vi "nanocal -- nuclear schottky fit V7.vi"() -> ()   [LabVIEW 2021] (continued)
                  n129 = Generate User Event(user event=w300, event data cluster="interface: update circle fit plot" ("event data")) -> (user event out=w295:refnum<user-event>)  [unwired: 2 in, 1 out]
                  n130 = Generate User Event(user event=w295, event data cluster="interface: update curvature plot" ("event data")) -> ()  [unwired: 2 in, 2 out]
                }
              }
              n131 = call "nanocal -- gradient descent.vi"("# steps"="#grad steps", "action"=nanocal_--_gradient_descent_--_action."step", "newton pars"=w288, "parameter keys IN"=w289, "parameter Map IN"=w283, "factors Map IN"=w282) -> ("logarithmic derivatives OUT"=w284:dbl[], "step factors OUT"=w291:map{T2, dbl}, "R(ω) out"=w281:cdb[], "goodness OUT"=w271:dbl, "oscillations"=→"Plot: oscillations":cluster{"Array":i32[], "Array":dbl[]})  [unwired: 1 in]
              n132 = for {
                tunnel: w289 -> [w302] mode=indexing
                shift-right: [w306] -> _
                shift-left: w291 -> [w306]
                shift-right: [w304] -> w272
                shift-left: w283 -> [w305]
                n133 = Look In Map(map=w306, key=w302) -> (value=w303:dbl)  [unwired: 1 in, 1 out]
                n134 = in-place {
                  in-place-border: w303 -> [w308]
                  n135 = in-place-map #1(w305, w302) -> (w309:dbl)  [unwired: 1 in, 1 out]
                  n136 = Multiply(x=w308, y=w309) -> (x*y=w307:dbl)
                  n137 = in-place-map #1(w307) -> (w304:map{T2, dbl})  [unwired: 1 in, 2 out]
                }
              }
              n138 = Absolute Value(x=w284) -> (abs(x)=→"|v_i| = | dlogG/dlogα_i | (log scale slider)":dbl[])
              n139 = local write "vector v=dlogG/dlogα of logarithmic derivatives"(w284) -> ()
              n140 = local write "R(ω) fit out"(w281) -> ()
              n141 = local write "Goodness"(w271) -> ()
              n142 = local write "parameter map"(w272) -> ()
              "current step ind" <- w275
            }
            n143 = local write "newton is active"(w263) -> ()
            "current  ind" <- 0 ("plot ind")
          }
          frame "action: parse string" {
            n144 = local read "String"() -> (w323:string)
            n145 = Generate User Event(user event=w315, event data cluster="interface: update list from parameter map" ("event data")) -> ()  [unwired: 2 in, 2 out]
            n146 = call "string parse mathematica assosiated array.vi"("action"=mathematica_string_map_action."parse string" ("derivative"), "String in"=w323) -> ("Map OUT"=w317:map{T2, dbl})  [unwired: 8 in, 1 out]
            n147 = Generate User Event ("action User Event")(user event=w321, event data cluster="action: update state of selectors" ("event data")) -> (user event out=w318:refnum<user-event>)  [unwired: 2 in, 1 out]
            n148 = Generate User Event ("action User Event")(user event=w318, event data cluster="action: replot colors" ("event data")) -> ()  [unwired: 2 in, 2 out]
            n149 = local write "parameter map"(w317) -> ()
          }
          frame "action: read mathematica string" {
            w333 = map{string, path} {}  # Size: 0
            w348 = map{T2, dbl} {}  # Size: 0
            w345 = set{dbl} {}  # Size: 0
            w349 = map{string, map{T2, dbl}} {}  # Size: 0
            w339 = map{string, string} {}  # Size: 0
            n150 = local read "side map to STR"() -> (w341:map{T8, string})
            n151 = local read "side map to NUM"() -> (w340:map{T8, i32})
            n152 = local read "data file parameters map"() -> (w342:map{T2, T18})
            n153 = local read "file pattern"() -> (w336:string)
            n154 = local read "folder"() -> (w337:path)
            n155 = Generate User Event(user event=w346, event data cluster="action: update enums" ("event data")) -> ()  [unwired: 2 in, 2 out]
            n156 = call "string parse mathematica list assosiated array -- V2.vi"("action"=3-lorentzian-heat-response_action."parse string" ("derivative"), "string IN"="string IN") -> ("Map OUT"=w350:map{string, map{T2, dbl}})  [unwired: 8 in, 1 out]
            n157 = call <vilib>:"Recursive File List.vi"("pattern"=w336, "Continue Recursing on Error? (F)"=TRUE, "Folder Path"=w337) -> ("All Files in Dir"=w334:path[])  [unwired: 4 in, 4 out]
            n158 = for {
              tunnel: w334 -> [w358] mode=indexing
              shift-right: [w372] -> w324
              shift-left: w350 -> [w382]
              shift-right: [w369] -> w344
              shift-left: w339 -> [w381]
              shift-right: [w368] -> w343
              shift-left: w349 -> [w377]
              shift-right: [w379] -> w328
              shift-left: w345 -> [w371]
              shift-right: [w370] -> w327
              shift-left: w345 -> [w380]
              tunnel: w348 -> [w375]
              shift-right: [w365] -> w326
              shift-left: w345 -> [w378]
              shift-right: [w367] -> w329
              shift-left: w345 -> [w376]
              tunnel: w342 -> [w374]
              shift-right: [w366] -> w331
              shift-left: w345 -> [w373]
              tunnel: w340 -> [w363]
              tunnel: w341 -> [w362]
              shift-right: [w359] -> w338
              shift-left: w333 -> [w360]
              w361 = T8[] [enum."sam", enum."ref"] items=["sam", "ref"]
              n159 = Strip Path(path=w358) -> (name=w357:string)  [unwired: 1 out]
              n160 = call "filename-manage.vi"("filename-action"=filename-action."getIDStock", "file name IN"=w357) -> ("string OUT"=w364:string)  [unwired: 7 in, 2 out]
              n161 = for {
                tunnel: w374 -> [w408]
                tunnel: w357 -> [w385]
                tunnel: w364 -> [w397]
                shift-right: [w406] -> w372
                shift-left: w382 -> [w417]
                shift-right: [w412] -> w379
                shift-left: w371 -> [w405]
                shift-right: [w404] -> w370
                shift-left: w380 -> [w413]
                shift-right: [w398] -> w365
                shift-left: w378 -> [w411]
                shift-right: [w399] -> w367
                shift-left: w376 -> [w409]
                shift-right: [w400] -> w366
                shift-left: w373 -> [w407]
                shift-right: [w401] -> w368
                shift-left: w377 -> [w410]
                shift-right: [w402] -> w369
                shift-left: w381 -> [w416]
                tunnel: w363 -> [w390]
                tunnel: w375 -> [w395]
                tunnel: w362 -> [w392]
                tunnel: w361 -> [w389] mode=indexing
                shift-right: [w386] -> w359
                shift-left: w360 -> [w387]
                tunnel: w358 -> [w384]
                # "internal key"
                n162 = Look In Map(map=w392, key=w389) -> (value=w391:string)  [unwired: 1 in, 1 out]
                n163 = Look In Map(map=w390, key=w389) -> (value=w388:i32)  [unwired: 1 in, 1 out]
                n164 = Concatenate Strings(w397, w391) -> (w396:string)
                n165 = Insert Into Map(map in=w395, key=3-lorentzian-parameters."side (S|R)", value=w388) -> (map out=w394:map{T2, dbl})  [unwired: 2 out]
                n166 = for {
                  shift-right: [w423] -> w403
                  shift-left: w394 -> [w424]
                  tunnel: w408 -> [w422] mode=indexing
                  tunnel: w385 -> [w420]
                  n167 = Unbundle(w422) -> ("key"=w421:T2, "filename-action"=w419:T18)
                  n168 = call "filename-manage.vi"("filename-action"=w419, "file name IN"=w420) -> ("number OUT"=w418:dbl)  [unwired: 7 in, 2 out]
                  n169 = Insert Into Map(map in=w424, key=w421, value=w418) -> (map out=w423:map{T2, dbl})  [unwired: 2 out]
                }
                n170 = in-place {
                  in-place-border: [w466] -> w415
                  in-place-border: w403 -> [w465]
                  n171 = in-place-map #2(w417, w396) -> (w464:map{T2, dbl}, w466:bool)  [unwired: 1 in]
                  n172 = for {
                    tunnel: w465 -> [w472] mode=indexing
                    shift-right: [w470] -> w463
                    shift-left: w464 -> [w471]
                    n173 = Unbundle(w472) -> ("key"=w469:T2, "number OUT"=w468:dbl)
                    n174 = Insert Into Map(map in=w471, key=w469, value=w468) -> (map out=w470:map{T2, dbl})  [unwired: 2 out]
                  }
                  n175 = in-place-map #2(w463, LVMapReplaceAction."Modify Entry only if found" ("action")) -> (w406:map{string, map{T2, dbl}})  [unwired: 2 out]
                }
                n176 = Not(x=w415) -> (.not. x?=w414:bool)
                n177 = case shown="True" w414 {
                  tunnel: w416 -> [w432 w462]
                  tunnel: [w432 w461] -> w402
                  tunnel: w385 -> [_ w460]
                  tunnel: w396 -> [_ w434]
                  tunnel: w413 -> [w430 w459]
                  tunnel: [w430 w458] -> w404
                  tunnel: w405 -> [w431 w457]
                  tunnel: [w431 w456] -> w412
                  tunnel: [w428 w455] -> w398
                  tunnel: w411 -> [w428 w454]
                  tunnel: w403 -> [_ w439]
                  tunnel: w410 -> [w429 w453]
                  tunnel: [w429 w452] -> w401
                  tunnel: [w427 w451] -> w399
                  tunnel: w409 -> [w427 w450]
                  tunnel: [w426 w441] -> w400
                  tunnel: w407 -> [w426 w440]
                  tunnel: w387 -> [w425 w436]
                  tunnel: [w425 w435] -> w386
                  tunnel: w384 -> [_ w433]
                  frame False {
                  }
                  frame True {
                    n178 = Look In Map(map=w439, key=3-lorentzian-parameters."set of (B|T)") -> (value=w442:dbl)  [unwired: 1 in, 1 out]
                    n179 = Look In Map(map=w439, key=3-lorentzian-parameters."side (S|R)") -> (value=w448:dbl)  [unwired: 1 in, 1 out]
                    n180 = Look In Map(map=w439, key=3-lorentzian-parameters."T (K)") -> (value=w446:dbl)  [unwired: 1 in, 1 out]
                    n181 = Look In Map(map=w439, key=3-lorentzian-parameters."B (T)") -> (value=w438:dbl)  [unwired: 1 in, 1 out]
                    n182 = Look In Map(map=w439, key=3-lorentzian-parameters."θ (deg)") -> (value=w437:dbl)  [unwired: 1 in, 1 out]
                    n183 = Insert Into Set(10:w442, 11:w440) -> (3:w441:set{dbl})  [unwired: 1 out]
                    n184 = Insert Into Set(10:w448, 11:w450) -> (3:w451:set{dbl})  [unwired: 1 out]
                    n185 = Insert Into Set(10:w446, 11:w454) -> (3:w455:set{dbl})  [unwired: 1 out]
                    n186 = Insert Into Set(10:w438, 11:w459) -> (3:w458:set{dbl})  [unwired: 1 out]
                    n187 = Insert Into Set(10:w437, 11:w457) -> (3:w456:set{dbl})  [unwired: 1 out]
                    n188 = Insert Into Map(map in=w453, key=w434, value=w439) -> (map out=w452:map{string, map{T2, dbl}})  [unwired: 2 out]
                    n189 = Insert Into Map(map in=w462, key=w434, value=w460) -> (map out=w461:map{string, string})  [unwired: 2 out]
                    n190 = Insert Into Map(map in=w436, key=w434, value=w433) -> (map out=w435:map{string, path})  [unwired: 2 out]
                  }
                }
              }
            }
            "all short filenames" <- w344
            "temps&degs" <- w343
            "mathematica thing" <- w324
            "all full filenames" <- w338
            n191 = local read "selector"() -> (w332:T10)
            n192 = in-place {
              in-place-border: w331 -> [w356]
              in-place-border: w329 -> [w355]
              in-place-border: w328 -> [w352]
              in-place-border: w327 -> [w353]
              in-place-border: w326 -> [w354]
              n193 = in-place-cluster #3(w332) -> ()  [unwired: 5 out]
              n194 = in-place-cluster #3("lookup.all set of"=w356, "lookup.all sides"=w355, "lookup.all T's"=w354, "lookup.all B's"=w353, "lookup.all θ's"=w352) -> (w330:T10)
            }
            n195 = local write "selector"(w330) -> ()
          }
          frame "action: update default values" {
            w477 = map{T2, cluster{"ζ":dbl, "ζ":dbl}[]} {}  # Size: 0
            (unwired) map{string, map{T2, dbl}} {} ("Map OUT")
            w475 = map{T2, dbl[]} {}  # Size: 0
            n196 = call "string parse mathematica list assosiated array -- V2.vi"("action"=3-lorentzian-heat-response_action."parse string" ("derivative"), "string IN"="default values string") -> ("Map OUT"=w478:map{string, map{T2, dbl}})  [unwired: 8 in, 1 out]
            n197 = for {
              tunnel: w478 -> [w504] mode=indexing
              tunnel: w473 -> [w503]
              shift-right: [w501] -> w476
              shift-left: w477 -> [w500]
              n198 = Unbundle(w504) -> ("Map"=w502:map{T2, dbl})  [unwired: 1 out]
              n199 = for {
                tunnel: w503 -> [w512] mode=indexing
                tunnel: w502 -> [w511]
                shift-right: [w506] -> w501
                shift-left: w500 -> [w505]
                # "parameter"
                # "temperatures"
                n200 = Look In Map(map=w511, key=w512) -> (value=w508:dbl)  [unwired: 1 in, 1 out]
                n201 = Look In Map(map=w505, key=w512) -> (value=w514:cluster{"ζ":dbl, "ζ":dbl}[])  [unwired: 1 in, 1 out]
                n202 = Look In Map(map=w511, key=3-lorentzian-parameters."T (K)" ("Plost: sweep window")) -> (value=w509:dbl)  [unwired: 1 in, 1 out]
                n203 = Bundle("ζ"=w509, "ζ"=w508) -> (w507:cluster{"ζ":dbl, "ζ":dbl})  [unwired: 1 in]
                n204 = Build Array (concatenate)(w514, w507) -> (w513:cluster{"ζ":dbl, "ζ":dbl}[])
                n205 = Insert Into Map(map in=w505, key=w512, value=w513) -> (map out=w506:map{T2, cluster{"ζ":dbl, "ζ":dbl}[]})  [unwired: 2 out]
              }
            }
            n206 = for {
              tunnel: w476 -> [w493] mode=indexing
              shift-right: [w490] -> w474
              shift-left: w475 -> [w489]
              # "sorted temperastures"
              # "parameter"
              # "temperastures"
              n207 = Unbundle(w493) -> ("Plost: sweep window"=w487:T2, w492:cluster{"ζ":dbl, "ζ":dbl}[])
              n208 = for {
                tunnel: w492 -> [w499] mode=indexing
                tunnel: [w498] -> w491 mode=indexing
                tunnel: [w497] -> w484 mode=indexing
                n209 = Unbundle(w499) -> ("ζ"=w498:dbl, "ζ"=w497:dbl)
              }
              n210 = call "array - sorted inexes.vi"("x"=w491) -> ("index array"=w483:i32[], "sorted array"=w485:dbl[])  [unwired: 9 in]
              n211 = Insert Into Map(map in=w489, key=3-lorentzian-parameters."T (K)", value=w485) -> (map out=w488:map{T2, dbl[]})  [unwired: 2 out]
              n212 = for {
                tunnel: w484 -> [w496]
                tunnel: w483 -> [w495] mode=indexing
                tunnel: [w494] -> w482 mode=indexing
                n213 = Index Array(array=w496, index=w495) -> (element=w494:dbl)
              }
              n214 = Insert Into Map(map in=w488, key=w487, value=w482) -> (map out=w490:map{T2, dbl[]})  [unwired: 2 out]
            }
            n215 = disable-structure shown="Disabled" {
              frame Disabled {
                # "2 3 4 0 1"
                # "2 3 4 5 6"
                # "5 6 2 3 4"
                n216 = call "array - sorted inexes.vi"() -> ()  [unwired: 10 in, 2 out]
              }
              frame Enabled {
              }
            }
            n217 = call "nanocal -- defaut parameter manager -- V1.vi"("action"=nanocal_--_defaut_parameter_manager_action--_V1."update", "internal map"=w474) -> ()  [unwired: 9 in, 1 out]
          }
          frame "action: empty string from filelist" {
            n218 = local read "file pattern"() -> (w516:string)
            n219 = local read "folder"() -> (w517:path)
            n220 = call <vilib>:"Recursive File List.vi"("pattern"=w516, "Continue Recursing on Error? (F)"=TRUE, "Folder Path"=w517) -> ("All Files in Dir"=w515:path[])  [unwired: 4 in, 4 out]
            n221 = for {
              tunnel: [w522] -> w519 mode=concatenating
              tunnel: w515 -> [w527] mode=indexing
              w525 = T8[] [enum."ref", enum."sam"] items=["sam", "ref"]
              n222 = Strip Path(path=w527) -> (name=w526:string)  [unwired: 1 out]
              n223 = local read "side map to STR"() -> (w524:map{T8, string})
              n224 = call "filename-manage.vi"("filename-action"=filename-action."getIDStock", "file name IN"=w526) -> ("string OUT"=w523:string)  [unwired: 7 in, 2 out]
              n225 = for {
                tunnel: w525 -> [w532] mode=indexing
                tunnel: w524 -> [w533]
                tunnel: w523 -> [w531]
                tunnel: [w529] -> w522 mode=indexing
                n226 = Look In Map(map=w533, key=w532) -> (value=w530:string)  [unwired: 1 in, 1 out]
                n227 = Concatenate Strings(w531, w530) -> (w529:string)
              }
            }
            n228 = call "string parse mathematica list assosiated array -- V2.vi"("action"=3-lorentzian-heat-response_action."create emty string" ("derivative"), "array of IDs"=w519) -> ("string out"=w520:string)  [unwired: 8 in, 1 out]
            n229 = local write "string OUT"(w520) -> ()
          }
          frame "action: update enums" {
            w537 = map{string, string} {}  # Size: 0
            w543 = map{i32, string} {}  # Size: 0
            # "gives a key"
            n230 = local read "selector"() -> (w535:T10)
            n231 = local read "all short filenames"() -> (w538:map{string, string})
            n232 = in-place {
              w560 = map{i32, dbl} {}  # Size: 0
              w566 = map{i32, dbl} {}  # Size: 0
              w567 = map{i32, dbl} {}  # Size: 0
              w569 = map{i32, dbl} {}  # Size: 0
              w568 = map{i32, dbl} {}  # Size: 0
              n233 = in-place-cluster #4(w535) -> ("lookup.all set of"=w554:set{dbl}, "lookup.all sides"=w553:set{dbl}, "lookup.all T's"=w552:set{dbl}, "lookup.all θ's"=w551:set{dbl}, "lookup.all B's"=w550:set{dbl})  [unwired: 5 out]
              n234 = for {
                shift-right: [w573] -> w559
                shift-left: w560 -> [w574]
                tunnel: [w571] -> w561 mode=indexing
                tunnel: w554 -> [w570] mode=indexing
                i -> [w572]
                n235 = Number To Decimal String(number=w570) -> (decimal integer string=w571:string)  [unwired: 1 in]
                n236 = Insert Into Map(map in=w574, key=w572, value=w570) -> (map out=w573:map{i32, dbl})  [unwired: 2 out]
              }
              n237 = for {
                shift-right: [w584] -> w556
                shift-left: w567 -> [w585]
                tunnel: [w582] -> w563 mode=indexing
                tunnel: w552 -> [w581] mode=indexing
                i -> [w583]
                n238 = Number To Fractional String(number=w581, precision (6)=i16 3) -> (F-format string=w582:string)  [unwired: 2 in]
                n239 = Insert Into Map(map in=w585, key=w583, value=w581) -> (map out=w584:map{i32, dbl})  [unwired: 2 out]
              }
              n240 = property on="set (1T|2B)" class="Ring (strict)"("Strings []"=w561) -> ()  [unwired: 2 in, 2 out]
              n241 = property on="T (K)" class="Ring (strict)"("Strings []"=w563) -> ()  [unwired: 2 in, 2 out]
              n242 = for {
                shift-right: [w578] -> w558
                shift-left: w566 -> [w579]
                tunnel: [w576] -> w562 mode=indexing
                tunnel: w553 -> [w575] mode=indexing
                i -> [w577]
                n243 = Number To Decimal String(number=w575) -> (decimal integer string=w576:string)  [unwired: 1 in]
                n244 = Insert Into Map(map in=w579, key=w577, value=w575) -> (map out=w578:map{i32, dbl})  [unwired: 2 out]
              }
              n245 = for {
                shift-right: [w596] -> w555
                shift-left: w568 -> [w597]
                tunnel: [w594] -> w564 mode=indexing
                tunnel: w551 -> [w593] mode=indexing
                i -> [w595]
                n246 = Number To Fractional String(number=w593, precision (6)=i16 3) -> (F-format string=w594:string)  [unwired: 2 in]
                n247 = Insert Into Map(map in=w597, key=w595, value=w593) -> (map out=w596:map{i32, dbl})  [unwired: 2 out]
              }
              n248 = property on="side (8S|4R)" class="Ring (strict)"("Strings []"=w562) -> ()  [unwired: 2 in, 2 out]
              n249 = property on="θ (deg)" class="Ring (strict)"("Strings []"=w564) -> ()  [unwired: 2 in, 2 out]
              n250 = for {
                shift-right: [w590] -> w557
                shift-left: w569 -> [w591]
                tunnel: [w588] -> w565 mode=indexing
                tunnel: w550 -> [w587] mode=indexing
                i -> [w589]
                n251 = Number To Fractional String(number=w587, precision (6)=i16 3) -> (F-format string=w588:string)  [unwired: 2 in]
                n252 = Insert Into Map(map in=w591, key=w589, value=w587) -> (map out=w590:map{i32, dbl})  [unwired: 2 out]
              }
              n253 = property on="B (T)" class="Ring (strict)"("Strings []"=w565) -> ()  [unwired: 2 in, 2 out]
              n254 = in-place-cluster #4("lookup.all set of"=w554, "lookup.all sides"=w553, "lookup.all T's"=w552, "lookup.all θ's"=w551, "lookup.all B's"=w550, "lookup.set of lookup"=w559, "lookup.side lookup"=w558, "lookup.T lookup"=w556, "lookup.B lookup"=w557, "lookup.θ lookup"=w555) -> (w534:T10)
            }
            n255 = for {
              tunnel: w538 -> [w602] mode=indexing
              shift-right: [w600] -> w536
              shift-left: w537 -> [w601]
              n256 = Unbundle(w602) -> ("event data"=w598:string, "file pattern"=w599:string)
              n257 = Insert Into Map(map in=w601, key=w599, value=w598) -> (map out=w600:map{string, string})  [unwired: 2 out]
            }
            n258 = local read "temps&degs"() -> (w542:map{string, map{T2, dbl}})
            n259 = local read "X selector"() -> (w541:T2)
            n260 = for {
              tunnel: [w611] -> w546 mode=indexing
              tunnel: [w615] -> w544 mode=indexing
              tunnel: [w612] -> w548 mode=indexing
              tunnel: w541 -> [w616]
              tunnel: w536 -> [w614] mode=indexing
              tunnel: w542 -> [w613]
              n261 = Unbundle(w614) -> (w611:string, w612:string)
              n262 = Look In Map(map=w613, key=w612) -> (value=w617:map{T2, dbl})  [unwired: 1 in, 1 out]
              n263 = Look In Map(map=w617, key=w616) -> (value=w615:dbl)  [unwired: 1 in, 1 out]
            }
            n264 = call "array - sorted inexes.vi"("x"=w544) -> ("index array"=w545:i32[])  [unwired: 9 in, 1 out]
            n265 = for {
              tunnel: w545 -> [w607] mode=indexing
              tunnel: w546 -> [w610]
              tunnel: [w609] -> w547 mode=indexing
              tunnel: w548 -> [w608]
              shift-right: [w603] -> w549
              shift-left: w543 -> [w606]
              i -> [w605]
              n266 = Index Array(array=w610, index=w607) -> (element=w609:string)
              n267 = Index Array(array=w608, index=w607) -> (element=w604:string)
              n268 = Insert Into Map(map in=w606, key=w605, value=w604) -> (map out=w603:map{i32, string})  [unwired: 2 out]
            }
            "filesnames lookup" <- w549
            n269 = property on="filenames" class="Ring (strict)"("Strings []"=w547) -> ()  [unwired: 2 in, 2 out]
            n270 = Generate User Event(user event=w539, event data cluster="action: update state of selectors" ("event data")) -> ()  [unwired: 2 in, 2 out]
            n271 = local write "selector"(w534) -> ()
          }
          frame "action: update constrained file selector" {
            w624 = map{i32, string} {}  # Size: 0
            n272 = local read "state of all selectors"() -> (w620:map{T2, map{bool, dbl}})
            n273 = local read "all short filenames"() -> (w621:map{string, string})
            n274 = local read "temps&degs"() -> (w622:map{string, map{T2, dbl}})
            n275 = for {
              tunnel: w621 -> [w634] mode=indexing
              tunnel: [w634] -> w623 mode=indexing if=w630
              shift-right: [w633] -> w619
              shift-left: w622 -> [w633]
              tunnel: w620 -> [w631]
              n276 = for {
                tunnel: [w646] -> w632 mode=indexing
                shift-right: [w641] -> _
                shift-left: w634 -> [w641]
                shift-right: [w640] -> _
                shift-left: w633 -> [w640]
                tunnel: w631 -> [w639] mode=indexing
                n277 = Unbundle(w641) -> ("event data"=w645:string)  [unwired: 1 out]
                n278 = Unbundle(w639) -> ("Plost: sweep window"=w638:T2, "map"=w637:map{bool, dbl})
                n279 = for {
                  tunnel: w637 -> [w649] mode=indexing
                  tunnel: [w648] -> w635
                  tunnel: [w647] -> w636
                  n280 = Unbundle(w649) -> ("ignore side !"=w648:bool, "number OUT"=w647:dbl)
                }
                n281 = Look In Map(map=w640, key=w645) -> (value=w644:map{T2, dbl})  [unwired: 1 in, 1 out]
                n282 = Look In Map(map=w644, key=w638) -> (value=w643:dbl)  [unwired: 1 in, 1 out]
                n283 = Equal?(x=w643, y=w636) -> (x = y?=w642:bool)
                n284 = Or(x=w635, y=w642) -> (x .or. y?=w646:bool)
              }
              n285 = And Array Elements(Boolean array=w632) -> (logical AND=w630:bool)
            }
            n286 = for {
              tunnel: [w664] -> w627 mode=indexing
              tunnel: [w662] -> w625 mode=indexing
              tunnel: [w659] -> w629 mode=indexing
              tunnel: w623 -> [w661] mode=indexing
              tunnel: w619 -> [w660]
              n287 = Unbundle(w661) -> ("event data"=w659:string, "file pattern"=w664:string)
              n288 = local read "X selector"() -> (w658:T2)
              n289 = Look In Map(map=w660, key=w659) -> (value=w663:map{T2, dbl})  [unwired: 1 in, 1 out]
              n290 = Look In Map(map=w663, key=w658) -> (value=w662:dbl)  [unwired: 1 in, 1 out]
            }
            n291 = call "array - sorted inexes.vi"("x"=w625) -> ("index array"=w626:i32[])  [unwired: 9 in, 1 out]
            n292 = for {
              tunnel: w626 -> [w654] mode=indexing
              tunnel: w627 -> [w657]
              tunnel: [w656] -> w628 mode=indexing
              tunnel: w629 -> [w655]
              shift-right: [w650] -> w618
              shift-left: w624 -> [w653]
              i -> [w652]
              n293 = Index Array(array=w657, index=w654) -> (element=w656:string)
              n294 = Index Array(array=w655, index=w654) -> (element=w651:string)
              n295 = Insert Into Map(map in=w653, key=w652, value=w651) -> (map out=w650:map{i32, string})  [unwired: 2 out]
            }
            "constrained filename lookup" <- w618
            n296 = property on="selection :|\\" class="Ring (strict)"("Strings []"=w628) -> ()  [unwired: 2 in, 2 out]
          }
          frame "action: constrained filenames select" {
            (unwired) 1
            n297 = local read "constrained filename lookup"() -> (w667:map{i32, string})
            n298 = local read "selection :|\\"() -> (w668:u16)
            n299 = local read "all full filenames"() -> (w669:map{string, path})
            n300 = Look In Map(map=w667, key=w668) -> (value=w670:string)  [unwired: 1 in, 1 out]
            n301 = Look In Map(map=w669, key=w670) -> (value=w671:path)  [unwired: 1 in, 1 out]
            n302 = local write "Read from file"(w671) -> ()
            n303 = Generate User Event(user event=w666, event data cluster="action: read from file" ("event data")) -> ()  [unwired: 2 in, 2 out]
          }
          frame "action: write mathematica string" {
            n304 = local read "mathematica thing"() -> (w676:map{string, map{T2, dbl}})
            n305 = local read "folder"() -> (w675:path)
            n306 = Build Path(base path=w675, name or relative path="temporarystring.txt") -> (appended path=w674:path)
            n307 = call "string parse mathematica list assosiated array -- V2.vi"("action"=3-lorentzian-heat-response_action."create string" ("derivative"), "Map IN"=w676) -> ("string out"=w672:string)  [unwired: 8 in, 1 out]
            "string OUT" <- w672
            n308 = Write to Text File(file (use dialog)=w674, text=w672) -> ()  [unwired: 2 in, 3 out]
          }
          frame "action: replot colors" {
            # "all -- including kappa0"
            n309 = local read "state of all selectors string"() -> (w687:string)
            n310 = local read "new selector names"() -> (w692:map{T2, map{T19, string}})
            n311 = local read "X selector"() -> (w688:T2)
            n312 = Build Array (concatenate)(w680, w678) -> (w679:T2[])
            n313 = local read "state of all selectors"() -> (w699:map{T2, map{bool, dbl}})
            n314 = Look In Map(map=w692, key=w688) -> (value=w691:map{T19, string})  [unwired: 1 in, 1 out]
            n315 = local read "mathematica thing"() -> (w700:map{string, map{T2, dbl}})
            n316 = Look In Map(map=w691, key=nameformattingitem."nameL") -> (value=w689:string)  [unwired: 1 in, 1 out]
            n317 = Concatenate Strings(w687, w689) -> (w698:string)
            n318 = for {
              tunnel: w700 -> [w721]
              tunnel: w688 -> [w716]
              tunnel: w679 -> [w704] mode=indexing
              tunnel: w699 -> [w717]
              tunnel: w692 -> [w708]
              shift-right: [w712] -> w686
              shift-left: w698 -> [w715]
              tunnel: w687 -> [w713]
              tunnel: [w709] -> w685 mode=indexing
              n319 = for {
                tunnel: w721 -> [w735] mode=indexing
                tunnel: w704 -> [w734]
                tunnel: [w733] -> w720 mode=indexing if=w727
                tunnel: [w732] -> w719 mode=indexing if=w727
                tunnel: w716 -> [w731]
                tunnel: w717 -> [w730]
                n320 = Unbundle(w735) -> ("Map"=w729:map{T2, dbl})  [unwired: 1 out]
                n321 = for {
                  tunnel: w730 -> [w744] mode=indexing
                  tunnel: w729 -> [w743]
                  tunnel: [w741] -> w728 mode=indexing
                  n322 = Unbundle(w744) -> ("Plost: sweep window"=w742:T2, "map"=w740:map{bool, dbl})
                  n323 = for {
                    tunnel: w740 -> [w747] mode=indexing
                    tunnel: [w746] -> w737
                    tunnel: [w745] -> w738
                    n324 = Unbundle(w747) -> ("ignore side !"=w746:bool, "number OUT"=w745:dbl)
                  }
                  n325 = Look In Map(map=w743, key=w742) -> (value=w739:dbl)  [unwired: 1 in, 1 out]
                  n326 = Equal?(x=w739, y=w738) -> (x = y?=w736:bool)
                  n327 = Or(x=w737, y=w736) -> (x .or. y?=w741:bool)
                }
                n328 = Look In Map(map=w729, key=w731) -> (value=w733:dbl)  [unwired: 1 in, 1 out]
                n329 = Look In Map(map=w729, key=w734) -> (value=w732:dbl)  [unwired: 1 in, 1 out]
                n330 = And Array Elements(Boolean array=w728) -> (logical AND=w727:bool)
              }
              n331 = Look In Map(map=w708, key=w704) -> (value=w706:map{T19, string})  [unwired: 1 in, 1 out]
              n332 = Look In Map(map=w706, key=nameformattingitem."nameL") -> (value=w705:string)  [unwired: 1 in, 1 out]
              n333 = call <vilib>:"Space Constant.vi"() -> ("String"=w714:string)
              n334 = Concatenate Strings(w715, w714, w713, w705) -> (w712:string)
              n335 = call "array - sorted inexes.vi"("x"=w720) -> ("index array"=w718:i32[])  [unwired: 9 in, 1 out]
              n336 = for {
                tunnel: w720 -> [w726]
                tunnel: w719 -> [w725]
                tunnel: w718 -> [w722] mode=indexing
                tunnel: [w724] -> w711 mode=indexing
                tunnel: [w723] -> w710 mode=indexing
                n337 = Index Array(array=w726, index=w722) -> (element=w724:dbl)
                n338 = Index Array(array=w725, index=w722) -> (element=w723:dbl)
              }
              n339 = Bundle(w711, w710) -> (w709:cluster{dbl[], dbl[]})  [unwired: 1 in]
            }
            n340 = local read "folder"() -> (w697:path)
            n341 = Concatenate Strings("plotstring", w687, ".dat") -> (w693:string)
            n342 = Build Path(base path=w697, name or relative path=w693) -> (appended path=w696:path)
            n343 = call "nanocal -- plotstring file manage.vi"("Enum"=nanocal_--_plotstring_file_action."generate plotstring thing", "all data"=w685, "header line"=w686) -> ("plotstring thing"=w683:string)  [unwired: 8 in]
            n344 = flat-sequence {
              tunnel: w685 -> [w701]
              tunnel: w682 -> [w703]
              tunnel: "interface: replot colors plot" ("event data") -> [w702]
              frame #0 {
                "color data" <- w701
              }
              frame #1 {
                n345 = Generate User Event(user event=w703, event data cluster=w702) -> ()  [unwired: 2 in, 2 out]
              }
            }
            n346 = Write to Text File(file (use dialog)=w696, text=w683) -> ()  [unwired: 2 in, 3 out]
          }
          frame "action: update state of selectors" {
            w768 = T2[] [enum."T (K)", enum."B (T)", enum."θ (deg)", enum."side (S|R)"] items=["ζ", "τ1", "τS", "τN", "τC", "κ0", "m1", "m2", "m3", "T (K)", "B (T)", "θ (deg)", "side (S|R)", "set of (B|T)", "Re(offset)", "Im(offset)", "στ1", "στ1-", "στ1+", "στS", "στS-", "στS+", "στN", "στN-", "στN+", "τ11", "τ12", "τ21", "τ22", "τN1", "τN2"]  # selector fields
            n347 = local read "selector"() -> (w764:T10)
            n348 = Unbundle By Name(w764) -> ("side (8S|4R)"=w763:i32, "ignore side !"=w762:bool, "lookup.side lookup"=w761:map{i32, dbl}, "T (K)"=w758:u16, "ignore T !"=w760:bool, "lookup.T lookup"=w759:map{i32, dbl}, "B (T)"=w755:u16, "ignore B !"=w757:bool, "lookup.B lookup"=w756:map{i32, dbl}, "θ (deg)"=w753:u16, "ignore θ !"=w752:bool, "lookup.θ lookup"=w754:map{i32, dbl}, "set (1T|2B)"=w749:i32, "ignore set of !"=w750:bool, "lookup.set of lookup"=w751:map{i32, dbl})
            n349 = Look In Map(map=w761, key=w763) -> (value=w767:dbl)  [unwired: 1 in, 1 out]
            n350 = local read "new selector names"() -> (w771:map{T2, map{T19, string}})
            n351 = node(w762, w767) -> (w788:map{bool, dbl})
            n352 = Look In Map(map=w759, key=w758) -> (value=w787:dbl)  [unwired: 1 in, 1 out]
            n353 = Look In Map(map=w756, key=w755) -> (value=w783:dbl)  [unwired: 1 in, 1 out]
            n354 = node(w760, w787) -> (w785:map{bool, dbl})
            n355 = node(w757, w783) -> (w782:map{bool, dbl})
            n356 = Look In Map(map=w754, key=w753) -> (value=w781:dbl)  [unwired: 1 in, 1 out]
            n357 = node(w752, w781) -> (w779:map{bool, dbl})
            n358 = Look In Map(map=w751, key=w749) -> (value=w778:dbl)  [unwired: 1 in, 1 out]
            n359 = node(w750, w778) -> (w776:map{bool, dbl})
            n360 = local read "side map from NUM"() -> (w765:map{i32, T8})
            n361 = node(3-lorentzian-parameters."side (S|R)" ("Plost: sweep window"), w788, 3-lorentzian-parameters."T (K)" ("Plost: sweep window"), w785, 3-lorentzian-parameters."B (T)" ("Plost: sweep window"), w782, 3-lorentzian-parameters."θ (deg)" ("Plost: sweep window"), w779, 3-lorentzian-parameters."set of (B|T)" ("Plost: sweep window"), w776) -> (w748:map{T2, map{bool, dbl}})
            "state of all selectors" <- w748
            n362 = for {
              tunnel: w771 -> [w793]
              shift-right: [w796] -> w769
              shift-left: "_" ("event data") -> [w795]
              tunnel: w768 -> [w792] mode=indexing
              tunnel: w748 -> [w790]
              n363 = Look In Map(map=w790, key=w792) -> (value=w798:map{bool, dbl})  [unwired: 1 in, 1 out]
              n364 = Look In Map(map=w793, key=w792) -> (value=w791:map{T19, string})  [unwired: 1 in, 1 out]
              n365 = for {
                tunnel: w798 -> [w813] mode=indexing
                tunnel: [w812] -> w797
                tunnel: [w811] -> w794
                n366 = Unbundle(w813) -> ("ignore side !"=w812:bool, "number OUT"=w811:dbl)
              }
              n367 = case shown="False" w797 {
                tunnel: [w809 w810] -> w796
                tunnel: w795 -> [w808 w810]
                tunnel: w794 -> [w805 _]
                tunnel: w791 -> [w801 _]
                frame False {
                  n368 = Look In Map(map=w801, key=nameformattingitem."units") -> (value=w802:string)  [unwired: 1 in, 1 out]
                  n369 = Look In Map(map=w801, key=nameformattingitem."prec") -> (value=w799:string)  [unwired: 1 in, 1 out]
                  n370 = Format Value(format string=w799, value (0)=w805) -> (output string=w804:string)  [unwired: 1 in]
                  n371 = Concatenate Strings(w808, "_" ("event data"), w804, w802, "_" ("event data")) -> (w809:string)
                }
                frame True {
                }
              }
            }
            "state of all selectors string" <- w769
            n372 = Look In Map(map=w765, key=w767) -> (value=w766:T8)  [unwired: 1 in, 1 out]
            n373 = local write "side"(w766) -> ()
            n374 = Generate User Event(user event=w772, event data cluster="action: replot colors" ("event data")) -> (user event out=w773:refnum<user-event>)  [unwired: 2 in, 1 out]
            n375 = Generate User Event(user event=w773, event data cluster="action: update constrained file selector" ("event data")) -> ()  [unwired: 2 in, 2 out]
          }
          frame "action: copy from math" {
            w823 = map{T2, bool} {}  # Size: 0
            n376 = local read "defaults selector"() -> (w822:T9)
            n377 = local read "mathematica thing"() -> (w828:map{string, map{T2, dbl}})
            n378 = case shown="True" "overwrite offset" {
              tunnel: w820 -> [w831 w835]
              tunnel: [w831 w834] -> w819
              frame False {
              }
              frame True {
                n379 = Build Array (concatenate)(w835, 3-lorentzian-parameters."Re(offset)" ("Plost: sweep window"), 3-lorentzian-parameters."Im(offset)" ("Plost: sweep window")) -> (w834:T2[])
              }
            }
            n380 = for {
              shift-right: [w839] -> w821
              shift-left: w823 -> [w840]
              tunnel: w822 -> [w838] mode=indexing
              n381 = Unbundle(w838) -> ("Plost: sweep window"=w837:T2, "used default"=w836:bool)
              n382 = Insert Into Map(map in=w840, key=w837, value=w836) -> (map out=w839:map{T2, bool})  [unwired: 2 out]
            }
            n383 = local read "key"() -> (w827:string)
            n384 = local read "parameter map"() -> (w816:map{T2, dbl})
            n385 = Look In Map(map=w828, key=w827) -> (key not found?=w825:bool, value=w826:map{T2, dbl})  [unwired: 1 in]
            n386 = case shown="False" w825 {
              tunnel: w826 -> [w855 _]
              tunnel: w821 -> [w853 _]
              tunnel: w819 -> [w854 _]
              tunnel: "overwrite offset" -> [w847 w892]
              tunnel: [w846 w892] -> w817
              tunnel: w816 -> [w845 _]
              tunnel: w814 -> [w843 _]
              frame False {
                # "the order of numbers \nMUST corrspond to order\nin the \"parameter\" array"
                n387 = for {
                  tunnel: [w867] -> w852 mode=indexing
                  tunnel: w855 -> [w875]
                  tunnel: w854 -> [w868] mode=indexing
                  tunnel: w853 -> [w874]
                  shift-right: [w869] -> w844
                  shift-left: w845 -> [w870]
                  n388 = Look In Map(map=w874, key=w868, default value=FALSE) -> (value=w873:bool)  [unwired: 1 out]
                  n389 = Look In Map(map=w875, key=w868) -> (value=w872:dbl)  [unwired: 1 in, 1 out]
                  n390 = case shown="True" w873 {
                    tunnel: w872 -> [w878 _]
                    tunnel: w868 -> [_ w879]
                    tunnel: [w878 w880] -> w867
                    frame False {
                    }
                    frame True {
                      n391 = local read "T (K)"() -> (w891:dbl)
                      n392 = local read "B (T)"() -> (w887:dbl)
                      n393 = Divide(x=w887, y=12.0) -> (x/y=w885:dbl)
                      n394 = Equal?(x=3-lorentzian-parameters."τN", y=w879) -> (x = y?=w888:bool)
                      n395 = Square(x=w885) -> (x^2=w884:dbl)
                      n396 = call "nanocal -- defaut parameter manager -- V1.vi"("action"=nanocal_--_defaut_parameter_manager_action--_V1."get logarithmic interp", "T"=w891, "what"=w879) -> ("number"=w882:dbl)  [unwired: 8 in]
                      n397 = Select(t=w884, s=w888, f=1.0) -> (s? t:f=w881:dbl)
                      n398 = Multiply(x=w882, y=w881) -> (x*y=w880:dbl)
                    }
                  }
                  n399 = in-place {
                    in-place-border: w867 -> [w877]
                    in-place-border: LVMapReplaceAction."Modify Entry only if found" ("action") -> [w876]
                    n400 = in-place-map #5(w870, w868) -> ()  [unwired: 1 in, 2 out]
                    n401 = in-place-map #5(w877, w876) -> (w869:map{T2, dbl})  [unwired: 2 out]
                  }
                }
                n402 = Index Array(array=w852, index #1=6 ("index"), index #2=7 ("index")) -> (element #1=w849:dbl, element #2=w848:dbl)
                n403 = flat-sequence {
                  tunnel: w844 -> [w856]
                  tunnel: w843 -> [w860]
                  tunnel: "interface: update list from parameter map" ("event data") -> [w859]
                  tunnel: "interface: update curvature plot" ("event data") -> [w857]
                  frame #0 {
                    n404 = local write "parameter map"(w856) -> ()
                  }
                  frame #1 {
                    n405 = Generate User Event(user event=w860, event data cluster=w859) -> (user event out=w858:refnum<user-event>)  [unwired: 2 in, 1 out]
                    n406 = Generate User Event(user event=w858, event data cluster=w857) -> ()  [unwired: 2 in, 2 out]
                  }
                }
                n407 = case shown="True" w847 {
                  selector: w847 -> [w861 w862]
                  tunnel: w849 -> [_ w864]
                  tunnel: w848 -> [_ w863]
                  tunnel: [w861 w862] -> w846
                  frame False {
                  }
                  frame True {
                    n408 = Bundle("number"=w864, "number"=w863) -> (w865:cluster{"number":dbl, "number":dbl})  [unwired: 1 in]
                    n409 = local write "offset Re\noffset Im"(w865) -> ()
                  }
                }
              }
              frame True {
              }
            }
            n410 = case shown="True" w817 {
              tunnel: ["action: new sweep" ("event data") "action: read from file" ("event data")] -> w815
              frame False {
              }
              frame True {
              }
            }
            n411 = Generate User Event(user event=w824, event data cluster=w815) -> ()  [unwired: 2 in, 2 out]
          }
          frame "action: copy to math" {
            n412 = local read "error goodness weighting"() -> (w904:T5)
            n413 = local read "offset Re\noffset Im"() -> (w915:cluster{"Numeric":dbl, "Numeric":dbl})
            n414 = local read "newton parameters"() -> (w906:T3)
            n415 = local read "sampling size(%)"() -> (w908:dbl)
            n416 = local read "curvature triplets"() -> (w910:T11[])
            n417 = local read "parameter map"() -> (w911:map{T2, dbl})
            n418 = local read "error-mode"() -> (w894:T15)
            n419 = call "nanocal -- publish -- freq scan V2.vi"("publisher action"=publisher_action."get") -> ("data"=w909:T34)  [unwired: 7 in, 3 out]
            n420 = local read "parameter map"() -> (w912:map{T2, dbl})
            n421 = local read "θ (deg)"() -> (w919:dbl)
            n422 = Build Array (concatenate)(w893, w896) -> (w895:T2[])
            n423 = local read "T (K)"() -> (w921:dbl)
            n424 = local read "B (T)"() -> (w920:dbl)
            n425 = Unbundle(w915) -> ("Numeric"=w914:dbl, "Numeric"=w913:dbl)
            n426 = Bundle By Name(cluster=w906, "weighting"=w904) -> (w905:T3)
            n427 = Generate User Event(user event=w925, event data cluster="action: replot colors" ("event data")) -> ()  [unwired: 2 in, 2 out]
            n428 = Build Array(w921, w920, w919, w914, w913) -> (w903:dbl[])
            n429 = call "nanocal -- generate 3D curvature ellipsoid --  V4.vi"("sampling vicinity size (%)"=w908, "error mode"=w894, "newton parameters"=w905, "data"=w909, "Curvature triplet array IN"=w910, "parameter map"=w911) -> ("Curvature triplet array OUT"=w900:T11[])  [unwired: 5 in]
            n430 = local write "curvature triplets"(w900) -> ()
            n431 = Index Array(array=w900, index=0) -> (element=w898:T11)
            n432 = Unbundle By Name(w898) -> ("pars & errors"=w897:map{T2, dbl})
            n433 = for {
              tunnel: w896 -> [w929] mode=indexing
              shift-right: [w930] -> _
              shift-left: w897 -> [w930]
              tunnel: [w928] -> w902 mode=indexing
              n434 = Look In Map(map=w930, key=w929, default value=0.0) -> (value=w928:dbl)  [unwired: 1 out]
            }
            n435 = Build Array (concatenate)(w903, w902) -> (w901:dbl[])
            n436 = for {
              tunnel: w901 -> [w931] mode=indexing
              tunnel: w895 -> [w932] mode=indexing
              shift-right: [w933] -> w918
              shift-left: w912 -> [w934]
              n437 = Insert Into Map(map in=w934, key=w932, value=w931) -> (map out=w933:map{T2, dbl})  [unwired: 2 out]
            }
            n438 = local read "mathematica thing"() -> (w924:map{string, map{T2, dbl}})
            n439 = local read "key"() -> (w923:string)
            n440 = call "3-lorentzian-heat-response -- V4.vi"("action"=3-lorentzian-heat-response_action."calc m1m2m3", "Map IN"=w918) -> ("Map OUT"=w917:map{T2, dbl})  [unwired: 7 in, 2 out]
            n441 = in-place {
              in-place-border: w917 -> [w935]
              n442 = in-place-map #6(w924, w923) -> (w938:map{T2, dbl})  [unwired: 1 in, 1 out]
              n443 = for {
                tunnel: w935 -> [w940] mode=indexing
                shift-right: [w943] -> w937
                shift-left: w938 -> [w944]
                shift-right: [w942] -> _
                shift-left: w935 -> [w942]
                n444 = Unbundle(w940) -> ("X selector"=w939:T2)  [unwired: 1 out]
                n445 = Look In Map(map=w942, key=w939) -> (value=w941:dbl)  [unwired: 1 in, 1 out]
                n446 = Insert Into Map(map in=w944, key=w939, value=w941) -> (map out=w943:map{T2, dbl})  [unwired: 2 out]
              }
              n447 = in-place-map #6(w937, LVMapReplaceAction."Modify Entry only if found" ("action")) -> (w922:map{string, map{T2, dbl}})  [unwired: 2 out]
            }
            n448 = local write "mathematica thing"(w922) -> ()
          }
          frame "action: exit" {
          }
          frame "action: read from file" {
            n449 = local read "Read from file"() -> (w946:path)
            n450 = local read "cursor x selector"() -> (w969:map{T2, dbl})
            n451 = call "file - read-write - list of lines-V2.vi"("read/write control"=file_--_read-write_control."read", "file path"=w946) -> ("header OUT"=w956:string, "list of lines OUT"=w958:string[], "filename out"=w986:string)  [unwired: 7 in]
            n452 = Unbundle("offset Re\noffset Im") -> ("Numeric"=w972:dbl, "Numeric"=w971:dbl)
            n453 = call "filename-manage.vi"("filename-action"=filename-action."get name", "file name IN"=w986) -> ("string OUT"=w955:string)  [unwired: 7 in, 2 out]
            n454 = Re/Im To Complex(1:w971, 2:w972) -> (0:w959:cdb)
            n455 = case shown="\"raw nanocal\"" "data file formatting" {
              tunnel: [w992 w1007 w1051 w1078] -> w980
              tunnel: [w991 w1006 w1050 w1077] -> w974
              tunnel: w959 -> [w990 w1015 w1046 w1067]
